vi "test-SwerveModuleState.vi"() -> ()   [LabVIEW 2019]
uses:
  <vilib>/Rock Robotics/WPI/ThirdParty/JAS_Junk/TrajLib/SWERVE_DRIVE_MODULE_STATE.ctl
  <vilib>/Rock Robotics/WPI/ThirdParty/JAS_Junk/TrajLib/ROTATION2D.ctl
  <vilib>/Rock Robotics/WPI/ThirdParty/JAS_Junk/TrajLib/Rotation_Minus.vi
  <vilib>/Rock Robotics/WPI/ThirdParty/JAS_Junk/TrajLib/Rotation_GetRadians.vi
  <vilib>/Rock Robotics/WPI/ThirdParty/JAS_Junk/TrajLib/Rotation_RotateBy.vi
  <vilib>/Rock Robotics/WPI/ThirdParty/JAS_Junk/TrajLib/Rotation_UnaryMinus.vi
  <vilib>/Rock Robotics/WPI/ThirdParty/JAS_Junk/TrajLib/Rotation_CreateXY.vi
  <vilib>/Rock Robotics/WPI/ThirdParty/JAS_Junk/TrajLib/Util_CalcDist.vi
  <vilib>/Rock Robotics/WPI/ThirdParty/JAS_Junk/TrajLib/Trajectory_Library.lvlib
panel:
  out "T91 Ang = reversed":T1={"Speed"=0.0, "Angle"={"VALUE"=0.0, "COS"=1.0, "SIN"=0.0}} {"Angle"."SIN" format="%13.4f"; "Angle"."COS" format="%13.4f"; "Angle"."VALUE" format="%13.4f"}
  out "T90  Ang = small":T1={"Speed"=0.0, "Angle"={"VALUE"=0.0, "COS"=1.0, "SIN"=0.0}} {"Angle"."SIN" format="%13.4f"; "Angle"."COS" format="%13.4f"; "Angle"."VALUE" format="%13.4f"}
  out "T3":T1={"Speed"=0.0, "Angle"={"VALUE"=0.0, "COS"=1.0, "SIN"=0.0}} {"Angle"."SIN" format="%13.4f"; "Angle"."COS" format="%13.4f"; "Angle"."VALUE" format="%13.4f"}
  out "T2":T1={"Speed"=0.0, "Angle"={"VALUE"=0.0, "COS"=1.0, "SIN"=0.0}} {"Angle"."SIN" format="%13.4f"; "Angle"."COS" format="%13.4f"; "Angle"."VALUE" format="%13.4f"}
  out "T1":i32
  out "T0":T1={"Speed"=0.0, "Angle"={"VALUE"=0.0, "COS"=1.0, "SIN"=0.0}} {"Angle"."SIN" format="%13.4f"; "Angle"."COS" format="%13.4f"; "Angle"."VALUE" format="%13.4f"}
  # "SwerveModuleState Test"
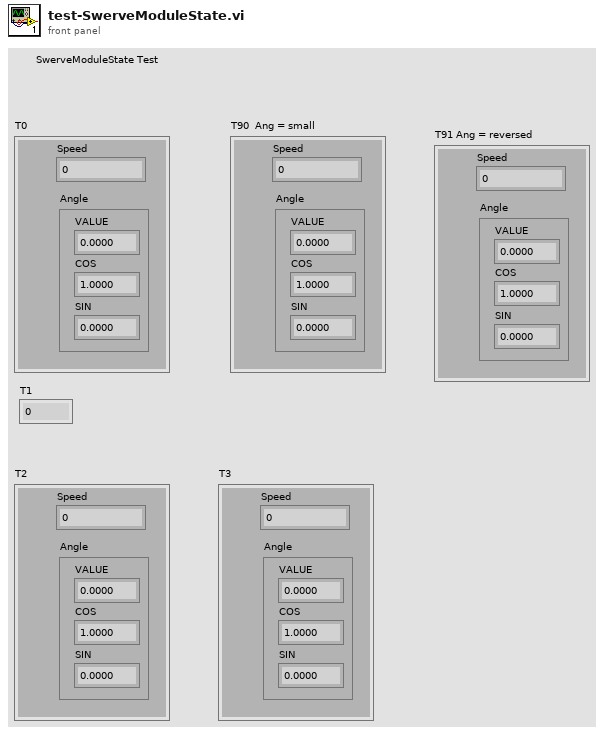
[diagram p1: front panel]
types:
  T1 = typedef "Trajectory_Library.lvlib/SWERVE_DRIVE_MODULE_STATE.ctl" = cluster{"Speed":dbl, "Angle":T2}
  T2 = typedef "Trajectory_Library.lvlib/ROTATION2D.ctl" = cluster{"VALUE":dbl, "COS":dbl, "SIN":dbl}
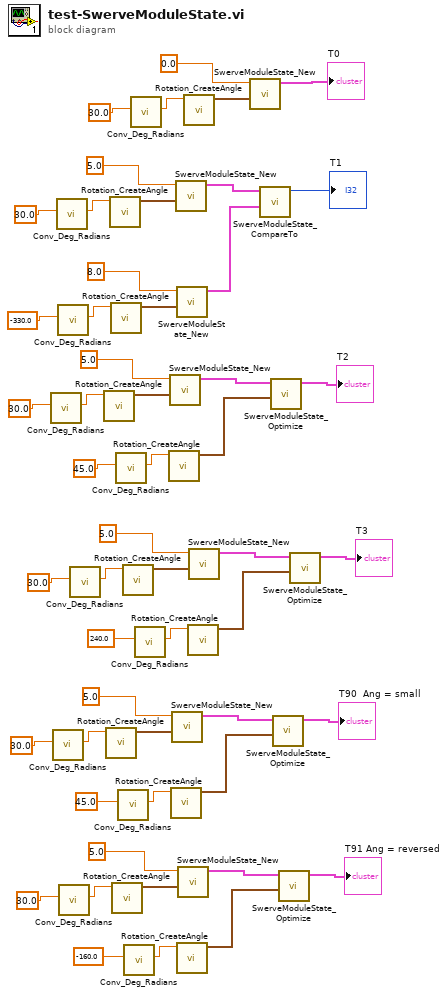
[diagram p0: block diagram]
diagram:
  n1 = call <vilib>:"Conv_Deg_Radians.vi"("Degress"=30.0 ("y")) -> ("Radians"=w36:dbl)  [unwired: 10 in]
  n2 = call <vilib>:"Conv_Deg_Radians.vi"("Degress"=30.0 ("y")) -> ("Radians"=w18:dbl)  [unwired: 10 in]
  n3 = call <vilib>:"Conv_Deg_Radians.vi"("Degress"=30.0 ("y")) -> ("Radians"=w47:dbl)  [unwired: 10 in]
  n4 = call <vilib>:"Conv_Deg_Radians.vi"("Degress"=-330.0 ("y")) -> ("Radians"=w43:dbl)  [unwired: 10 in]
  n5 = call <vilib>:"Conv_Deg_Radians.vi"("Degress"=30.0 ("y")) -> ("Radians"=w9:dbl)  [unwired: 10 in]
  n6 = call <vilib>:"Conv_Deg_Radians.vi"("Degress"=30.0 ("y")) -> ("Radians"=w27:dbl)  [unwired: 10 in]
  n7 = call <vilib>:"Rotation_CreateAngle.vi"("Angle"=w36) -> ("ROTATION"=w33:T2)  [unwired: 10 in]
  n8 = call <vilib>:"Rotation_CreateAngle.vi"("Angle"=w18) -> ("ROTATION"=w16:T2)  [unwired: 10 in]
  n9 = call <vilib>:"Rotation_CreateAngle.vi"("Angle"=w47) -> ("ROTATION"=w44:T2)  [unwired: 10 in]
  n10 = call <vilib>:"Rotation_CreateAngle.vi"("Angle"=w43) -> ("ROTATION"=w40:T2)  [unwired: 10 in]
  n11 = call <vilib>:"Rotation_CreateAngle.vi"("Angle"=w9) -> ("ROTATION"=w7:T2)  [unwired: 10 in]
  n12 = call <vilib>:"Conv_Deg_Radians.vi"("Degress"=45.0 ("y")) -> ("Radians"=w30:dbl)  [unwired: 10 in]
  n13 = call <vilib>:"Conv_Deg_Radians.vi"("Degress"=45.0 ("y")) -> ("Radians"=w13:dbl)  [unwired: 10 in]
  n14 = call <vilib>:"Rotation_CreateAngle.vi"("Angle"=w27) -> ("ROTATION"=w25:T2)  [unwired: 10 in]
  n15 = call <vilib>:"Conv_Deg_Radians.vi"("Degress"=-160.0 ("y")) -> ("Radians"=w4:dbl)  [unwired: 10 in]
  n16 = call <vilib>:"Conv_Deg_Radians.vi"("Degress"=30.0 ("y")) -> ("Radians"=w52:dbl)  [unwired: 10 in]
  n17 = call <vilib>:"Conv_Deg_Radians.vi"("Degress"=240.0 ("y")) -> ("Radians"=w22:dbl)  [unwired: 10 in]
  n18 = call <vilib>:"Rotation_CreateAngle.vi"("Angle"=w30) -> ("ROTATION"=w28:T2)  [unwired: 10 in]
  n19 = call <vilib>:"SwerveModuleState_New.vi"("ROTATION"=w33, "Speed"=5.0) -> ("SWERVE_DRIVE_MODULE_STATE"=w32:T1)  [unwired: 9 in]
  n20 = call <vilib>:"Rotation_CreateAngle.vi"("Angle"=w13) -> ("ROTATION"=w11:T2)  [unwired: 10 in]
  n21 = call <vilib>:"SwerveModuleState_New.vi"("ROTATION"=w16, "Speed"=5.0) -> ("SWERVE_DRIVE_MODULE_STATE"=w15:T1)  [unwired: 9 in]
  n22 = call <vilib>:"SwerveModuleState_New.vi"("ROTATION"=w44, "Speed"=5.0) -> ("SWERVE_DRIVE_MODULE_STATE"=w38:T1)  [unwired: 9 in]
  n23 = call <vilib>:"SwerveModuleState_New.vi"("ROTATION"=w40, "Speed"=8.0) -> ("SWERVE_DRIVE_MODULE_STATE"=w37:T1)  [unwired: 9 in]
  n24 = call <vilib>:"Rotation_CreateAngle.vi"("Angle"=w4) -> ("ROTATION"=w2:T2)  [unwired: 10 in]
  n25 = call <vilib>:"SwerveModuleState_New.vi"("ROTATION"=w7, "Speed"=5.0) -> ("SWERVE_DRIVE_MODULE_STATE"=w6:T1)  [unwired: 9 in]
  n26 = call <vilib>:"Rotation_CreateAngle.vi"("Angle"=w52) -> ("ROTATION"=w48:T2)  [unwired: 10 in]
  n27 = call <vilib>:"Rotation_CreateAngle.vi"("Angle"=w22) -> ("ROTATION"=w20:T2)  [unwired: 10 in]
  n28 = call <vilib>:"SwerveModuleState_New.vi"("ROTATION"=w25, "Speed"=5.0) -> ("SWERVE_DRIVE_MODULE_STATE"=w24:T1)  [unwired: 9 in]
  n29 = call <vilib>:"SwerveModuleState_New.vi"("ROTATION"=w48, "Speed"=0.0) -> ("SWERVE_DRIVE_MODULE_STATE"=→"T0":T1)  [unwired: 9 in]
  n30 = call <vilib>:"SwerveModuleState_CompareTo.vi"("other SWERVE_DRIVE_MODULE_STATE"=w37, "in SWERVE_DRIVE_MODULE_STATE"=w38) -> ("Compare"=→"T1":i32)  [unwired: 9 in]
  n31 = call <vilib>:"SwerveModuleState_Optimize.vi"("CurrentAngle"=w28, "Desired State"=w32) -> ("out SWERVE_DRIVE_MODULE_STATE"=→"T2":T1)  [unwired: 9 in]
  n32 = call <vilib>:"SwerveModuleState_Optimize.vi"("CurrentAngle"=w11, "Desired State"=w15) -> ("out SWERVE_DRIVE_MODULE_STATE"=→"T90  Ang = small":T1)  [unwired: 9 in]
  n33 = call <vilib>:"SwerveModuleState_Optimize.vi"("CurrentAngle"=w2, "Desired State"=w6) -> ("out SWERVE_DRIVE_MODULE_STATE"=→"T91 Ang = reversed":T1)  [unwired: 9 in]
  n34 = call <vilib>:"SwerveModuleState_Optimize.vi"("CurrentAngle"=w20, "Desired State"=w24) -> ("out SWERVE_DRIVE_MODULE_STATE"=→"T3":T1)  [unwired: 9 in]
